vi "Baseband Transmission-Simple .vi"() -> ()   [LabVIEW 2013]
uses:
  <vilib>/Analysis/2dsp.llb/1D Convolution (DBL).vi
  <vilib>/Analysis/2dsp.llb/Decimate (single shot, DBL).vi
  <vilib>/Analysis/2dsp.llb/Upsample (DBL).vi
  <vilib>/Analysis/NI_AALBase.lvlib
  <vilib>/Analysis/NI_AALPro.lvlib
panel:
  in  "Sinc Samples":i32=65
  out "Recovered Bits":i32[](array[numeric])
  in  "stop":bool
  in  "UpSample Factor":i32(slide)=74 scale=1.0..100.0
  out "Symbol":dbl[](array[numeric])
  in  "Bit":i32[](array[numeric])=[0, 0, 0, 1, 0, 1, 1, 1, 0, 0]
  in  "Pulse Shaping Function":enum16{"Triangle", "Sinc ", "Rcosine"}(ring)=enum."Sinc "
  out "Pulse Shaping":dbl[](graph)
  out "Baseband":dbl[](graph)
  # "Baseband Transmission"
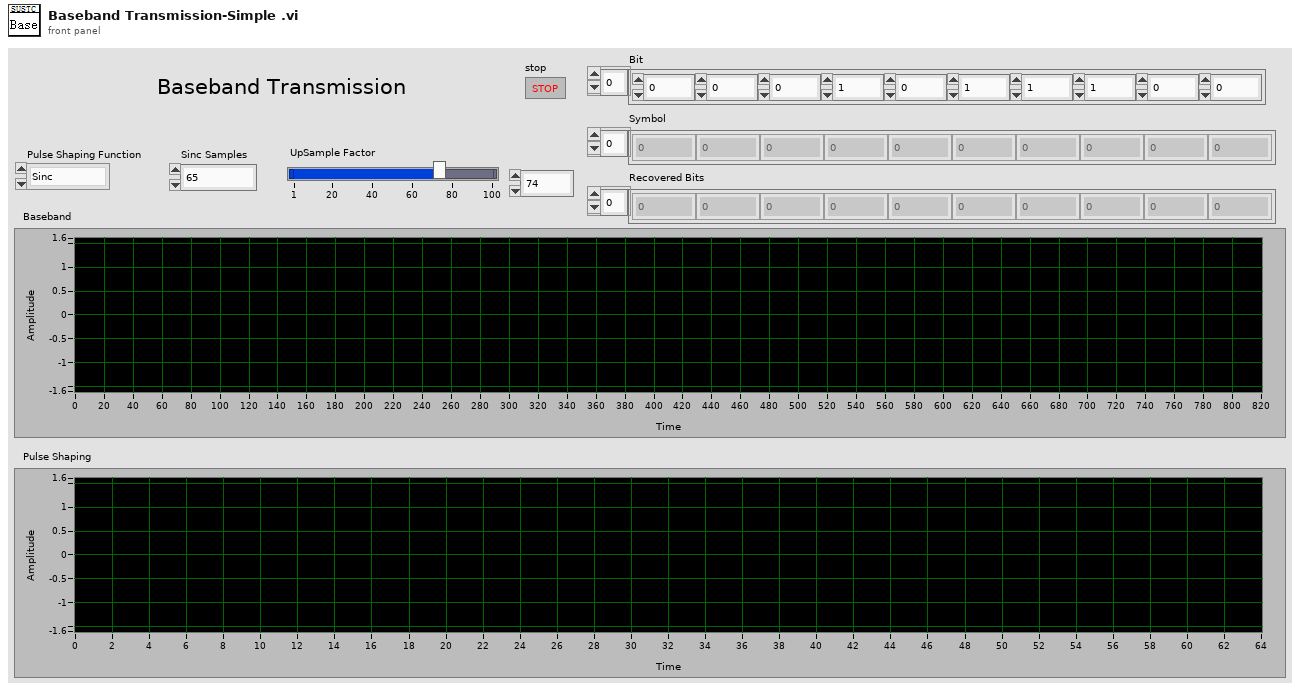
[diagram p1: front panel]
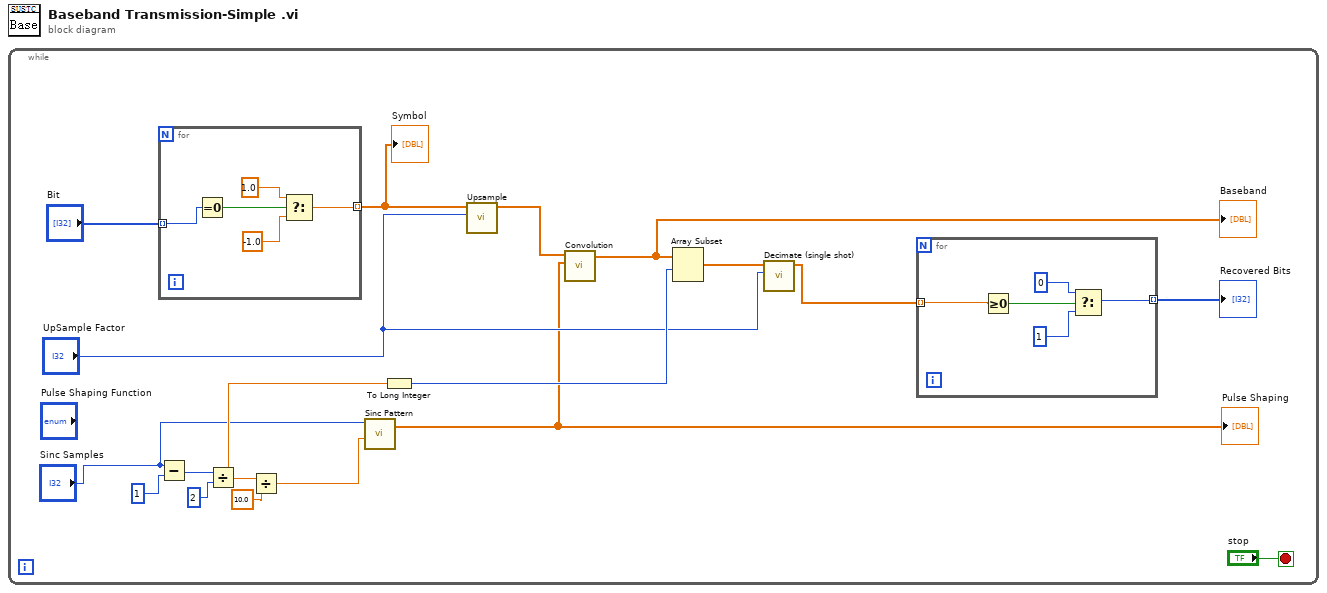
[diagram p0: block diagram]
diagram:
  n1 = while {
    stop <- "stop" stop-if-true
    n2 = for {
      tunnel: [w25] -> w7 mode=indexing
      tunnel: "Bit" -> [w24] mode=indexing
      n3 = Equal To 0?(x=w24) -> (x = 0?=w28:bool)
      n4 = Select(t=1.0, s=w28, f=-1.0) -> (s? t:f=w25:dbl)
    }
    "Symbol" <- w7
    n5 = Subtract(x="Sinc Samples", y=1) -> (x-y=w15:i32)
    n6 = Divide(x=w15, y=2) -> (x/y=w11:dbl)
    n7 = Divide(x=w11, y=10.0) -> (x/y=w12:dbl)
    n8 = call <vilib>:"Sinc Pattern.vi"("delay"=w12, "samples"="Sinc Samples") -> ("Sinc Pattern"=w1:dbl[])  [unwired: 2 in, 1 out]
    "Pulse Shaping" <- w1
    n9 = To Long Integer(number=w11) -> (32bit integer=w3:i32)
    n10 = call-poly <vilib>:"Upsample.vi"("upsampling factor"="UpSample Factor", "X"=w7) -> ("Upsampled Array"=w9:dbl[])  [unwired: 8 in, 1 out]
    n11 = call-poly <vilib>:"Convolution.vi"("Y"=w1, "X"=w9) -> ("X * Y"=w4:dbl[])  [unwired: 8 in, 1 out]
    "Baseband" <- w4
    n12 = Array Subset "Array Subset"(array=w4, index=w3) -> (w8:dbl[])  [unwired: 1 in]
    n13 = call-poly <vilib>:"Decimate (single shot).vi"("decimating factor"="UpSample Factor", "X"=w8) -> ("Decimated Array"=w6:dbl[])  [unwired: 8 in, 1 out]
    n14 = for {
      tunnel: w6 -> [w20] mode=indexing
      tunnel: [w21] -> w5 mode=indexing
      n15 = Greater Or Equal To 0?(x=w20) -> (x >= 0?=w19:bool)
      n16 = Select(t=0, s=w19, f=1) -> (s? t:f=w21:i32)
    }
    "Recovered Bits" <- w5
  }
